vi "Check Reentrancy Changes.vi"(8 "error in":errorcluster, 10 "Master VI Ref":refnum<vi>, 11 "File Info in":T1) -> (0 "error out":errorcluster, 3 "File Info out":T1)   [LabVIEW 2020, in "Peer Review.lvclass"]
uses:
  Peer Review.lvclass
  TypeDefs/File Info.ctl
  TypeDefs/File State.ctl
  TypeDefs/VI Type.ctl
  Peer Review.lvclass/Peer Review.ctl
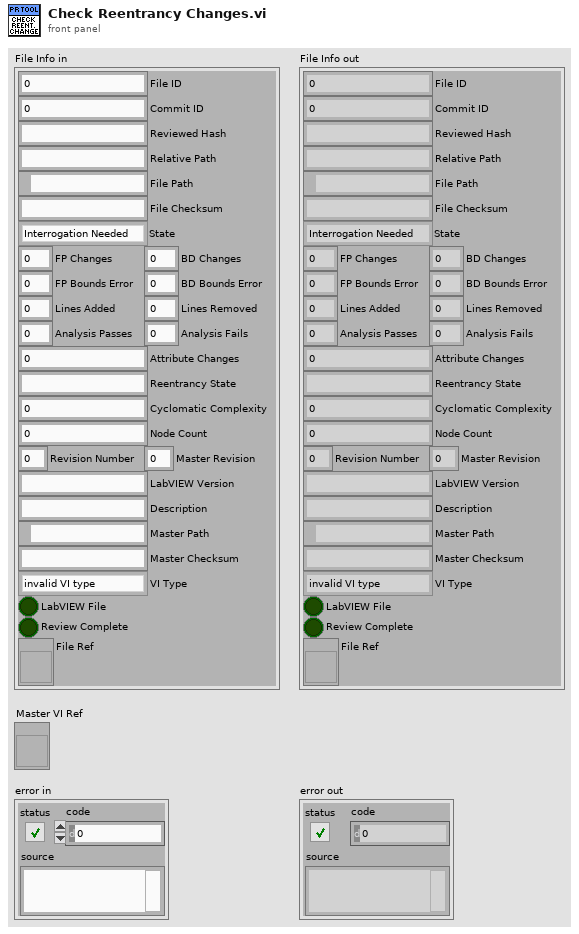
[diagram p1: front panel]
types:
  T1 = typedef "Peer Review.lvclass/File Info.ctl" = cluster{"File ID":i32, "Commit ID":i32, "Reviewed Hash":string, "Relative Path":string, "File Path":path, "File Checksum":string, "State":T2, "FP Changes":i32, "BD Changes":i32, "FP Bounds Error":dbl, "BD Bounds Error":dbl, "Lines Added":i32, "Lines Removed":i32, "Analysis Passes":i32, "Analysis Fails":i32, "Attribute Changes":i32, "Reentrancy State":string, "Cyclomatic Complexity":i32, "Node Count":i32, "Revision Number":u32, "LabVIEW Version":string, "Description":string, "Master Path":path, "Master Checksum":string, "VI Type":T3, "LabVIEW File":bool, "Review Complete":bool, "File Ref":refnum<vi>, "Master Revision":u32}
  T2 = typedef "Peer Review.lvclass/File State.ctl" = enum16{"Interrogation Needed", "Modified", "Deleted", "Added", "Matches Previous", "No Changes", "Moved", "Empty File"}
  T3 = typedef "Peer Review.lvclass/VI Type.ctl" = enum32{"invalid VI type", "Standard VI", "Control VI", "Global VI", "Polymorphic VI", "Configuration VI", "SubSystem", "Facade VI", "Method VI", "Statechart Diagram VI"}
  T4 = enum16{"Share clones between instances", "Preallocate clone for each instance"}
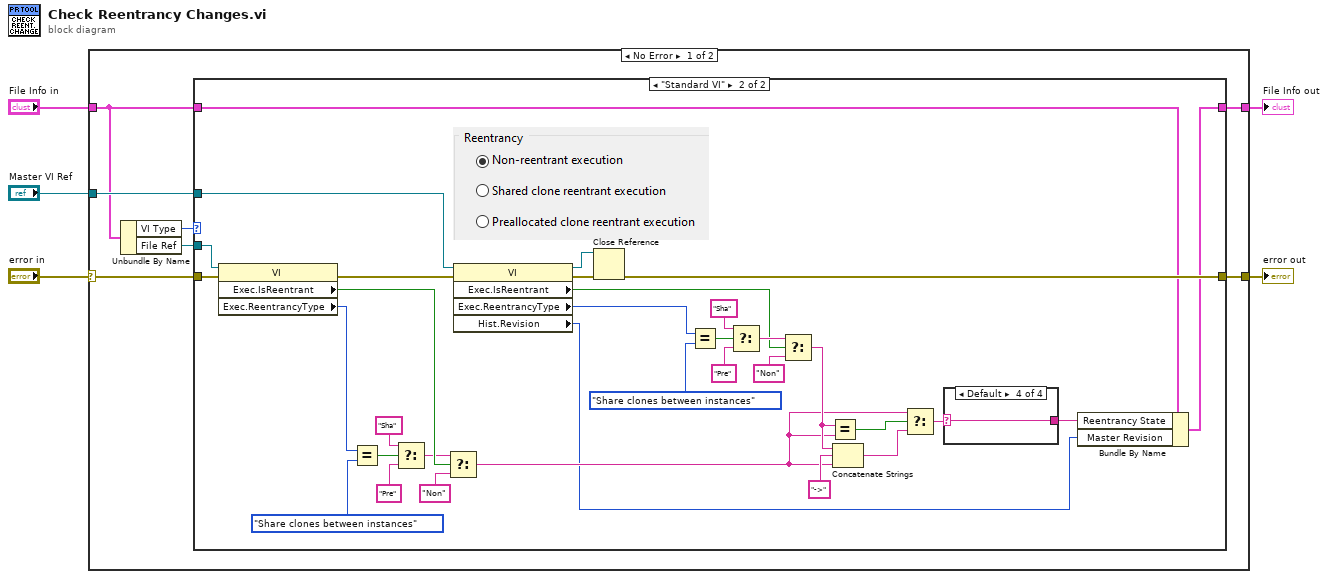
[diagram p0: block diagram]
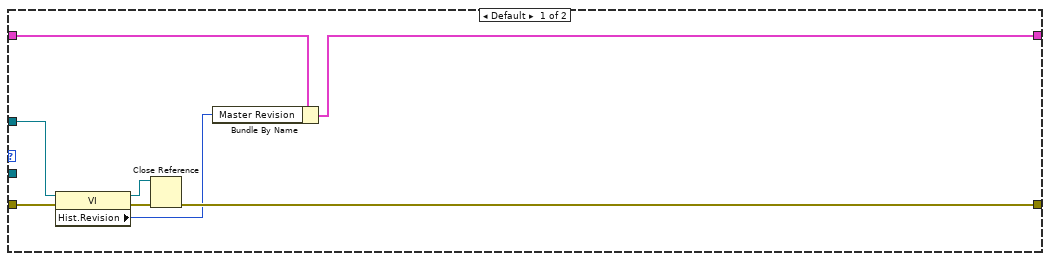
[diagram p2: hidden frame]
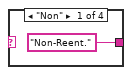
[diagram p3: hidden frame]
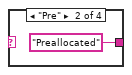
[diagram p4: hidden frame]
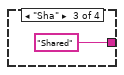
[diagram p5: hidden frame]
diagram:
  n1 = case shown="No Error" "error in" {
    selector: "error in" -> [w6 w59]
    tunnel: "Master VI Ref" -> [w12 _]
    tunnel: [w11 w59] -> w4
    tunnel: "File Info in" -> [w9 w58]
    tunnel: [w10 w58] -> w1
    frame No Error {
      n2 = Unbundle By Name(w9) -> ("VI Type"=w8:T3, "File Ref"=w7:refnum<vi>)
      n3 = case shown="\"Standard VI\"" w8 {
        tunnel: w12 -> [w18 w53]
        tunnel: [w20 w51] -> w11
        tunnel: w6 -> [w16 w49]
        tunnel: w7 -> [_ w48]
        tunnel: w9 -> [w15 w26]
        tunnel: [w14 w25] -> w10
        frame Default {
          n4 = property on="Property Node" class="VI"(reference=w18, error in=w16) -> (reference out=w19:refnum<vi>, error out=w17:errorcluster, "Hist.Revision"=w13:u32)
          n5 = Close Reference(reference=w19, error in (no error)=w17) -> (error out=w20:errorcluster)
          n6 = Bundle By Name(cluster=w15, "Master Revision"=w13) -> (w14:T1)
        }
        frame "Standard VI" {
          n7 = property on="Property Node" class="VI"(reference=w48, error in=w49) -> (error out=w47:errorcluster, "Exec.IsReentrant"=w43:bool, "Exec.ReentrancyType"=w46:T4)  [unwired: 1 out]
          n8 = Equal?(x=w46, y=T4."Share clones between instances") -> (x = y?=w44:bool)
          n9 = Select(t="Sha", s=w44, f="Pre") -> (s? t:f=w42:string)
          n10 = Select(t=w42, s=w43, f="Non") -> (s? t:f=w24:string)
          n11 = property on="Property Node" class="VI"(reference=w53, error in=w47) -> (reference out=w50:refnum<vi>, error out=w52:errorcluster, "Exec.IsReentrant"=w31:bool, "Exec.ReentrancyType"=w32:T4, "Hist.Revision"=w21:u32)
          n12 = Close Reference(reference=w50, error in (no error)=w52) -> (error out=w51:errorcluster)
          n13 = Equal?(x=w32, y=T4."Share clones between instances") -> (x = y?=w34:bool)
          n14 = Select(t="Sha", s=w34, f="Pre") -> (s? t:f=w35:string)
          n15 = Select(t=w35, s=w31, f="Non") -> (s? t:f=w30:string)
          n16 = Equal?(x=w30, y=w24) -> (x = y?=w28:bool)
          n17 = Concatenate Strings(w30, "->" ("string"), w24) -> (w27:string)
          n18 = Select(t=w24, s=w28, f=w27) -> (s? t:f=w23:string)
          n19 = case shown="Default" w23 {
            selector: w23 -> [_ _ _ w57]
            tunnel: ["Non-Reent." "Preallocated" "Shared" w57] -> w22
            frame "Non" {
            }
            frame "Pre" {
            }
            frame "Sha" {
            }
            frame Default {
            }
          }
          n20 = Bundle By Name(cluster=w26, "Reentrancy State"=w22, "Master Revision"=w21) -> (w25:T1)
        }
      }
    }
    frame Error {
    }
  }
  "error out" <- w4
  "File Info out" <- w1
